vi "Execute.vi"(8 "error in (no error)":errorcluster, 10 "Context in":refnum<class "Context.lvclass">, 11 "Full Force Test Command in":refnum<class "Sentran Accuracy Test Command.lvclass">) -> (0 "error out":errorcluster, 2 "Context out":refnum<class "Context.lvclass">, 3 "Full Force Test Command out":refnum<class "Sentran Accuracy Test Command.lvclass">)   [LabVIEW 2016, in "Sentran Accuracy Test Command.lvclass"]
uses:
  Sentran Accuracy Test Command.lvclass
  Context/Context.lvclass
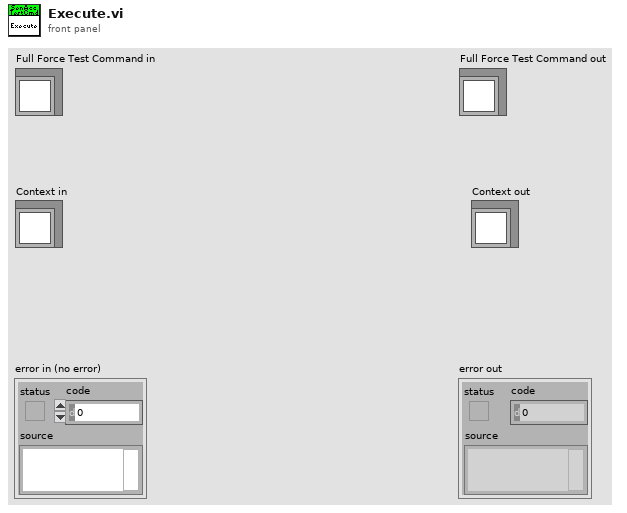
[diagram p1: front panel]
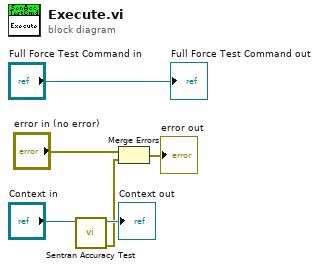
[diagram p0: block diagram]
diagram:
  n1 = call-dynamic "Sentran Accuracy Test.vi"("Context in"="Context in") -> ("error out"=w4:errorcluster, "Context out"=→"Context out":refnum<class "Context.lvclass">)  [unwired: 9 in]
  n2 = Merge Errors("error in (no error)", w4) -> (→"error out":errorcluster)
  "Full Force Test Command out" <- "Full Force Test Command in"
